vi "Map Poly to Pixels.vi"(9 "Draw Area Size":T1, 10 "Position":cluster{"Left":dbl, "Top":dbl}, 11 "Coords":cluster{"Horizontal":dbl, "Vertical":dbl}[](array[cluster])) -> (3 "Coords":cluster{"Horizontal":dbl, "Vertical":dbl}[](array[cluster]))   [LabVIEW 2020]
uses:
  <vilib>/Utility/miscctls.llb/LVBoundsTypeDef.ctl
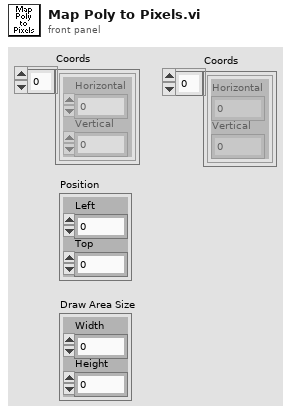
[diagram p1: front panel]
types:
  T1 = typedef "LVBoundsTypeDef.ctl" = cluster{"Width":u32, "Height":u32}
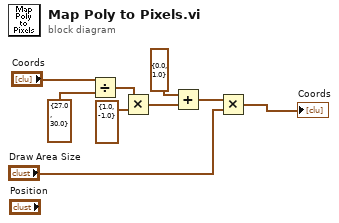
[diagram p0: block diagram]
diagram:
  n1 = Divide(x="Coords", y=cluster{"Width":dbl, "Height":dbl} {"Width"=27.0, "Height"=30.0} ("Bounds")) -> (x/y=w4:cluster{dbl, dbl}[])
  n2 = Multiply(x=w4, y=cluster{"Width":dbl, "Height":dbl} {"Width"=1.0, "Height"=-1.0} ("Bounds")) -> (x*y=w3:cluster{dbl, dbl}[])
  n3 = Add(x=cluster{"Width":dbl, "Height":dbl} {"Width"=0.0, "Height"=1.0} ("Bounds"), y=w3) -> (x+y=w2:cluster{dbl, dbl}[])
  n4 = Multiply(x=w2, y="Draw Area Size") -> (x*y=→"Coords":cluster{dbl, dbl}[])
